vi "Text control 2 v0.1.vi"() -> ()   [LabVIEW 2013]
panel:
  out "Ion vs time":cluster{"Y data in":dbl[], "X data in":dbl[]}[](graph)
  out "Ig":dbl format="%.2e"
  out "Id":dbl format="%.2e"
  out "Is":dbl format="%.2e"
  out "I vs Vg":cluster{"Y data in":dbl[], "X data in":dbl[]}[](graph)
  in  "Suffix":string=".txt"
  in  "Prefix":string="-transfer-"
  in  "Panel Controls 2":T1={"Emergency Stop"=refnum, "TransGraph Max"=1e-05, "Text/Graph (text=false)"=TRUE, "TransGraph Min"=1e-11} {"TransGraph Min" format="%.2e"; "TransGraph Max" format="%.2e"}
  out "Currently running:":string="#output s 0 0 0 -0.008 0.008 0.002"
  in  "Lines left to run:":string
  in  "Standby":T2
  in  "Full Reset":bool
  in  "SMU4":cluster{"on/off":bool, "Voltage":dbl} {"Voltage" min=-100.0 max=100.0 format="%.2f"}
  in  "Source/Drain\nRange":u8(slide)=6 max=11 scale=0.0..11.0
  in  "Source/Drain\nRange mode":u16(ring) items=["Auto", "Limited", "Fixed"]
  in  "Gate Range":u8(slide)=6 max=11 scale=0.0..11.0
  in  "Gate Range\nmode":u16(ring) items=["Auto", "Limited", "Fixed"]
  in  "Gate":T3={"Gate Start"=0.0, "Gate Stop"=2.0, "Gate Step (linear only)"=1.0, "Gate Compliance"=0.0001, "Gate PComp"=0.0, "Range mode"=0, "Range"=6} {"Range" max=11 scale=0.0..11.0; "Range mode" items=["Auto", "Limited", "Fixed"]; "Gate PComp" format="%^.2e"; "Gate Compliance" format="%^.2e"; "Gate Step (linear only)" format="%^.4e"; "Gate Stop" format="%^.4e"; "Gate Start" format="%^.4e"}
  in  "Drain 2":T4={"Drain Start"=0.0, "Drain Stop"=2.0, "Drain Compliance"=0.0001, "Drain Step"=1.0, "Drain PComp"=0.0, "Range mode"=0, "Range"=6} {"Range" max=11 scale=0.0..11.0; "Range mode" items=["Auto", "Limited", "Fixed"]; "Drain PComp" format="%^.2e"; "Drain Step" format="%^.4e"; "Drain Compliance" format="%^.2e"; "Drain Stop" format="%^.4e"; "Drain Start" format="%^.4e"}
  in  "Timings 2":T5={"integration time"=0, "Short/Long integration time"=0.00064, "hold time (sec)"=0.0, "delay time (sec)"=0.0, "Step Time (0 disables)"=0.0, "sweep method"=0, "Pulse period"=0.005, "Base voltage"=0.0, "Pulse width"=0.0005} {"Pulse width" min=0.0005 max=0.1 step=0.0001 format="%.4f"; "Base voltage" format="%^.4e"; "Pulse period" min=0.005 max=1.0 step=0.0001 format="%.4f"; "sweep method" items=["Continuous", "Pulsed"]; "Step Time (0 disables)" format="%.2f"; "delay time (sec)" format="%.4f"; "hold time (sec)" format="%.4f"; "Short/Long integration time" format="%^.0e"; "integration time" scale=0.0..2.0}
  in  "Panel Controls":T6={"Emergency Stop"=refnum, "TransGraph Max"=1e-05, "Text/Graph (text=false)"=TRUE} {"TransGraph Max" format="%.2e"}
  in  "Interrupt run":bool
  in  "Drain: Compliance":dbl=0.001 format="%.8f"
  in  "Gate: Compliance":dbl=0.001 format="%.8f"
  out "Path":path=path "C:/users/rlp38/09Apr2009LTtesting/test2.txt"
  in  "hold time /s":dbl format="%.2f"
  in  "delay time /s":dbl format="%.2f"
  in  "integration time":u32(slide) max=2 step=1 scale=0.0..2.0
  in  "Integration time (short)":dbl=0.0019 min=8e-05 max=0.0019 step=8e-05 format="%^.0e"
  in  "Integration time (long)":dbl=0.32 min=0.04 max=2.0 step=0.02 format="%.2f"
  in  "Step delay /s":dbl format="%.2f"
  in  "Program":string="#pulsedstressV d 0.03 20 0 0.5 0.0827 5\n#\n#itime m\n#gaterangemode a\n#drainrangemode a\n#pulsed on 0.05 0 0.02\n#transfer d -10 40 1 5 40 35\n#transfer d -10 40 1 5 40 35\n#transfer d -10 40 1 5 40 35\n#output d 0 40 20 0 40 1\n#\n#\n#sample 1 0.008 221 6 0.003\n#samplei 400e-6 200 6 0.002 0.1\n#vsu2pulse -10 4\n#\n#stressV 0.016 0.03 2e-4 0.1e-3 11\n#stressI 220e-7 0.08 15\n#transfer s -1 1 0.5 -0.005 0.005 0.005\n#output s 0 0 0 -0.008 0.008 0.002\n"
  # "Syntax:\nitime [s|m|l]\ngaterangemode [a|l|f]\ndrainrangemode [a|l|f]\npulsed [on|off] PulsePeriod(sec) PulseBaseVoltage PulseONWidth(sec)\nstandby [on l off]\nwait NumMilliseconds\nwait-min NumMinutes\n# texthere = comment\ntransfer [s|d] VgStart VgStop VgStep VdStart VdStop VdStep\noutput [s|d] VgStart VgStop VgStep VdStart VdStop VdStep\nsample Vg Vd NumSamples Time(s) SampleInterval(s)\nsamplei Idg NumSamples Time(s) SampleInterval(s) VDGcompliance\n# if in doubt use SampleInterval(s) = 0.004\nstressV VG VD IGcompliance IDcompliance Duration(sec)\nstressI IDG VDGcompliance Duration(sec)\nvsu2pulse Bias Duration(s)\npulsedstressV [s|d] VEstop VgON VgOFF Period(s) PulseONwidth(s) Vd\nsample-fpp Vg Vd NumSamples Time\nresample-fpp Vg Vd\ntransfer-fpp [s|d] VgStart VgStop VgStep VdStart VdStop VdStep\noutput-fpp [s|d] VgStart VgStop VgStep VdStart VdStop VdStep"
  # "100 samples is approx 13s with medium integration"
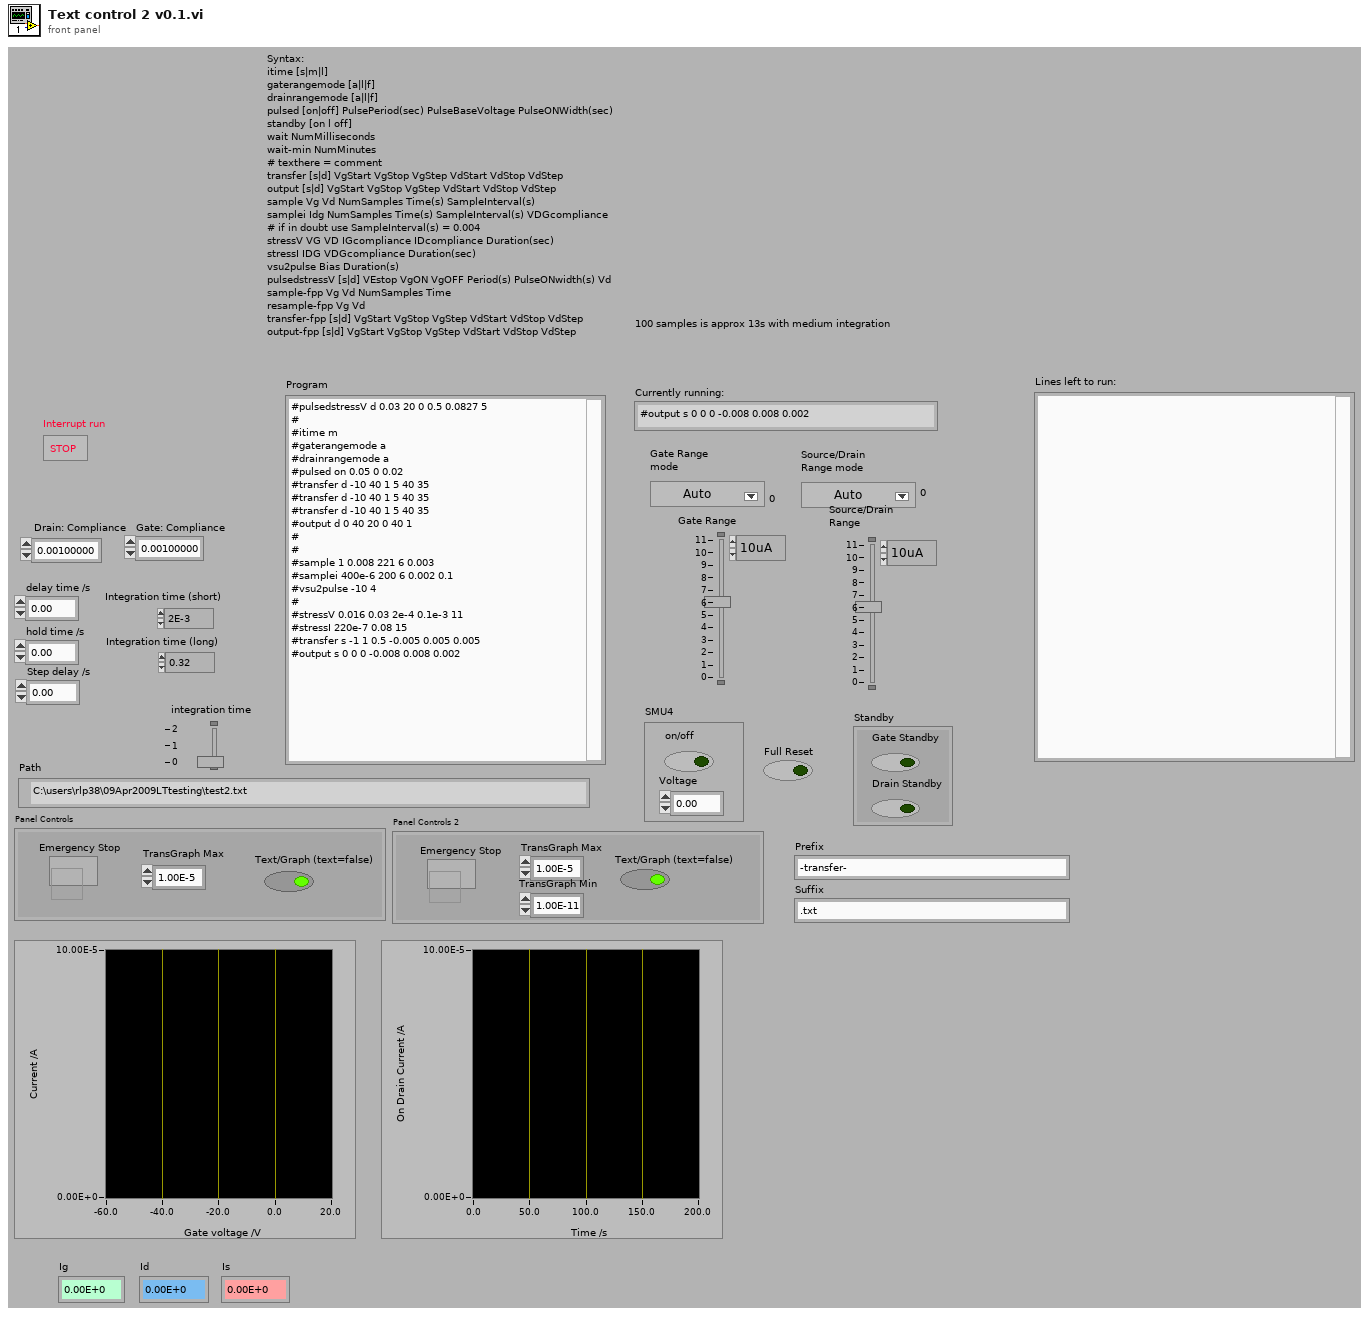
[diagram p1: front panel]
types:
  T1 = cluster{"Emergency Stop":refnum<vi>, "TransGraph Max":dbl, "Text/Graph (text=false)":bool, "TransGraph Min":dbl}
  T2 = cluster{"Gate Standby":bool, "Drain Standby":bool}
  T3 = cluster{"Gate Start":dbl, "Gate Stop":dbl, "Gate Step (linear only)":dbl, "Gate Compliance":dbl, "Gate PComp":dbl, "Range mode":u16, "Range":u8}
  T4 = cluster{"Drain Start":dbl, "Drain Stop":dbl, "Drain Compliance":dbl, "Drain Step":dbl, "Drain PComp":dbl, "Range mode":u16, "Range":u8}
  T5 = cluster{"integration time":u32, "Short/Long integration time":dbl, "hold time (sec)":dbl, "delay time (sec)":dbl, "Step Time (0 disables)":dbl, "sweep method":u16, "Pulse period":dbl, "Base voltage":dbl, "Pulse width":dbl}
  T6 = cluster{"Emergency Stop":refnum<vi>, "TransGraph Max":dbl, "Text/Graph (text=false)":bool}
  T7 = enum16{"open", "replace", "create", "open or create", "replace or create", "replace or create with confirmation"}
  T8 = cluster{"V2 Start":dbl, "V2 Step":dbl, "Number of points":i32}
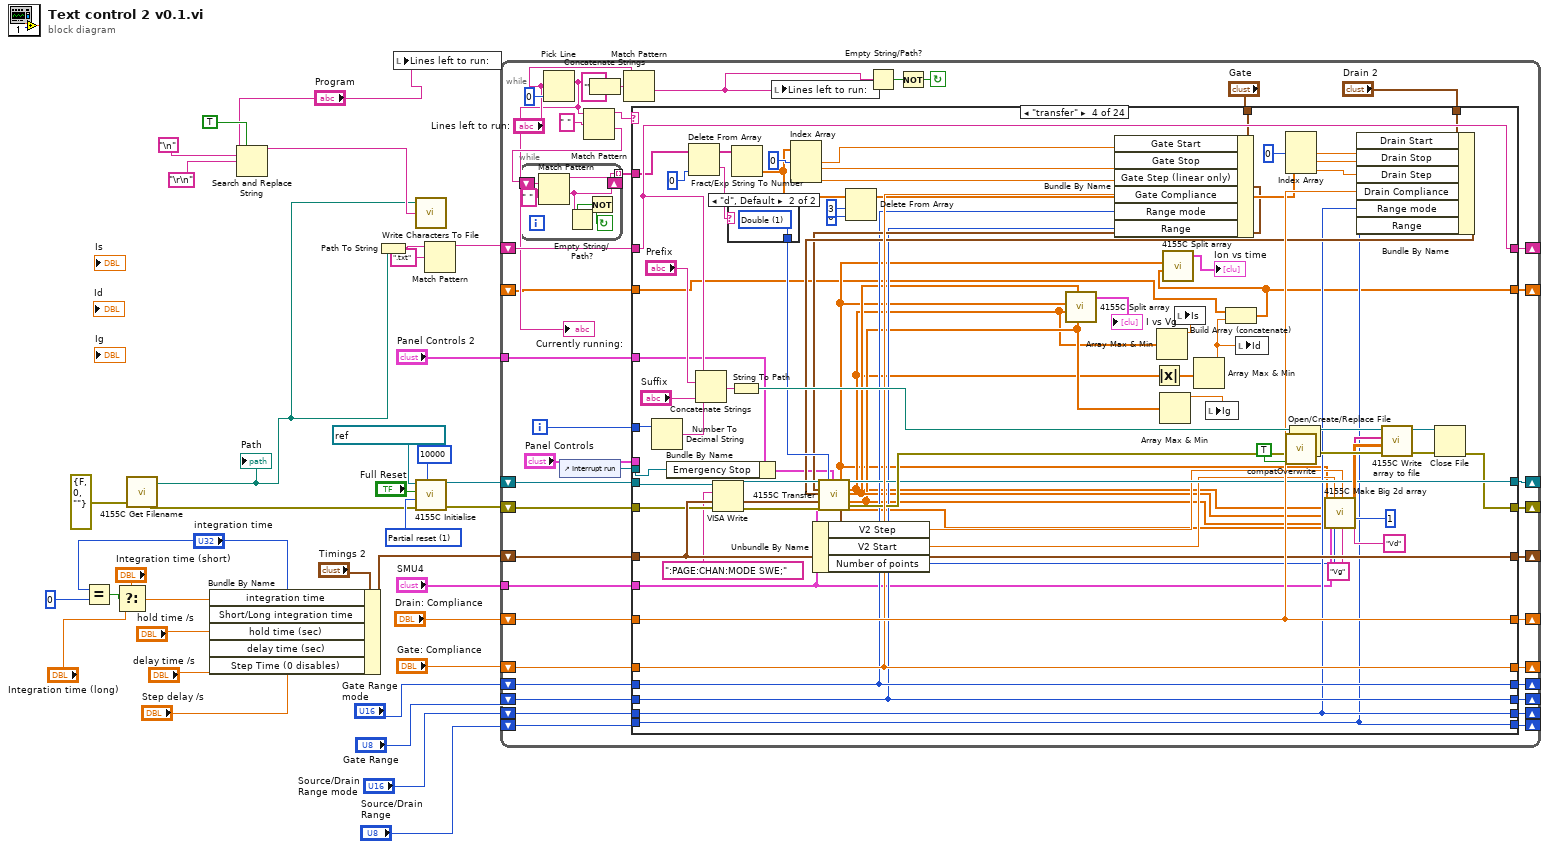
[diagram p0: block diagram]
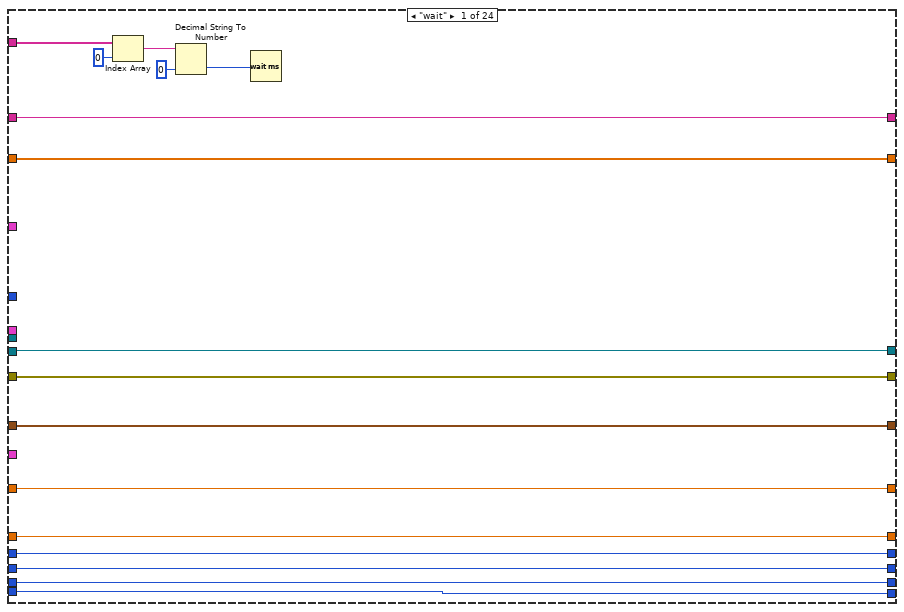
[diagram p2: hidden frame]
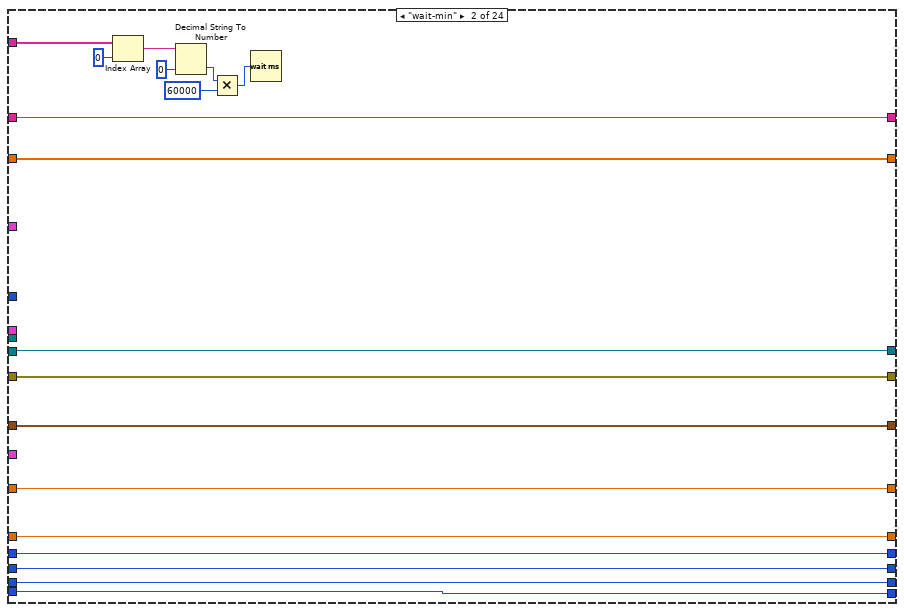
[diagram p3: hidden frame]
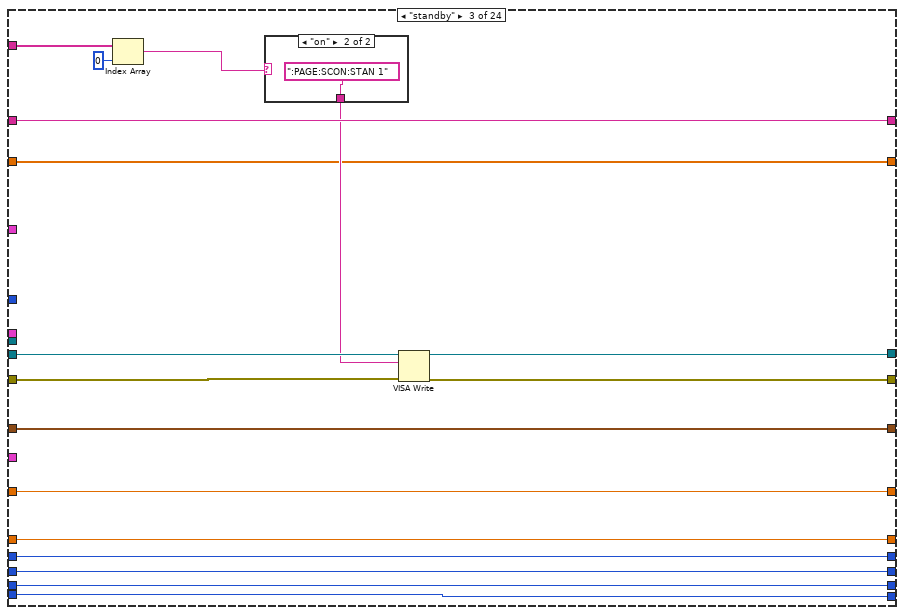
[diagram p4: hidden frame]
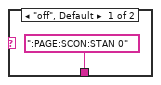
[diagram p5: hidden frame]
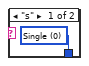
[diagram p6: hidden frame]
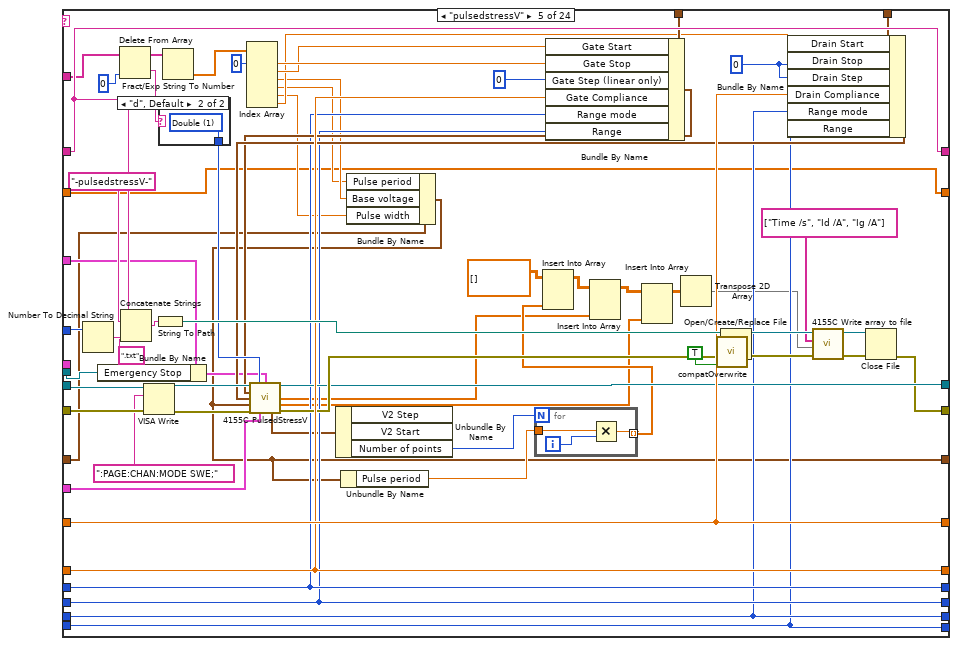
[diagram p7: hidden frame]
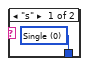
[diagram p8: hidden frame]
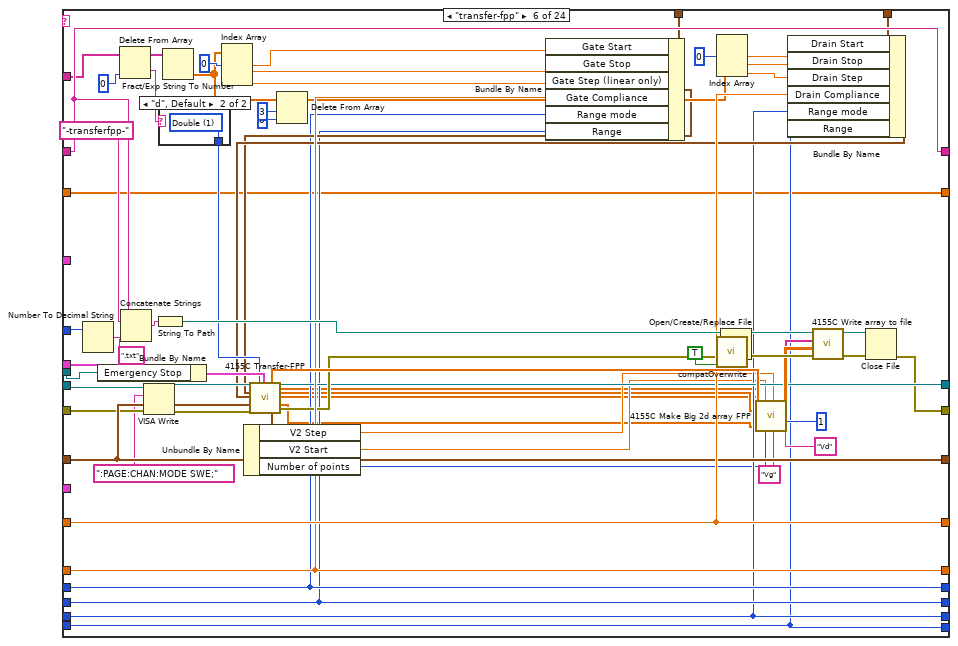
[diagram p9: hidden frame]
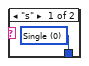
[diagram p10: hidden frame]
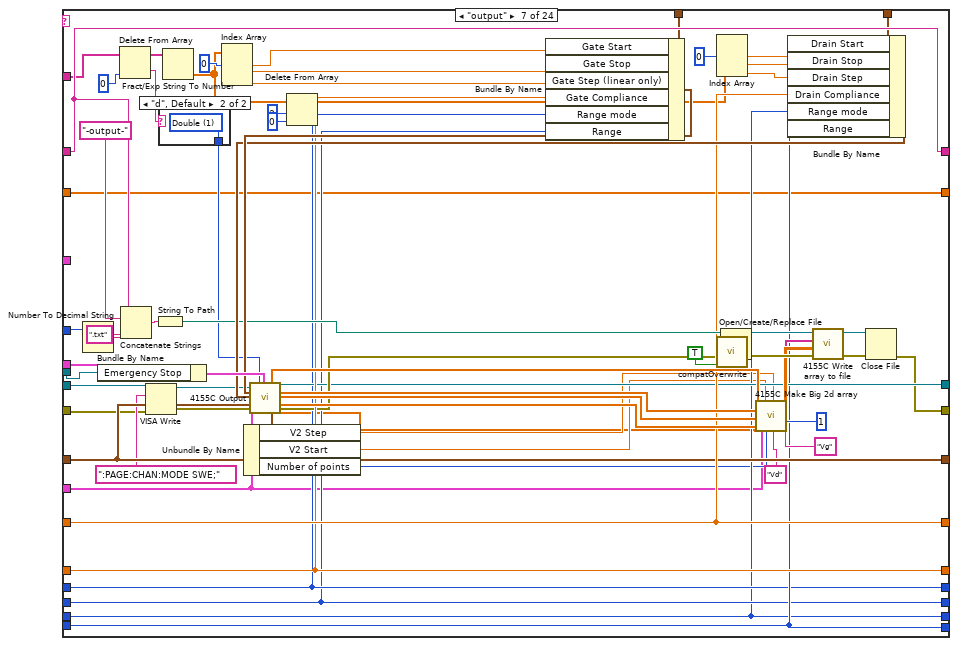
[diagram p11: hidden frame]
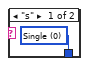
[diagram p12: hidden frame]
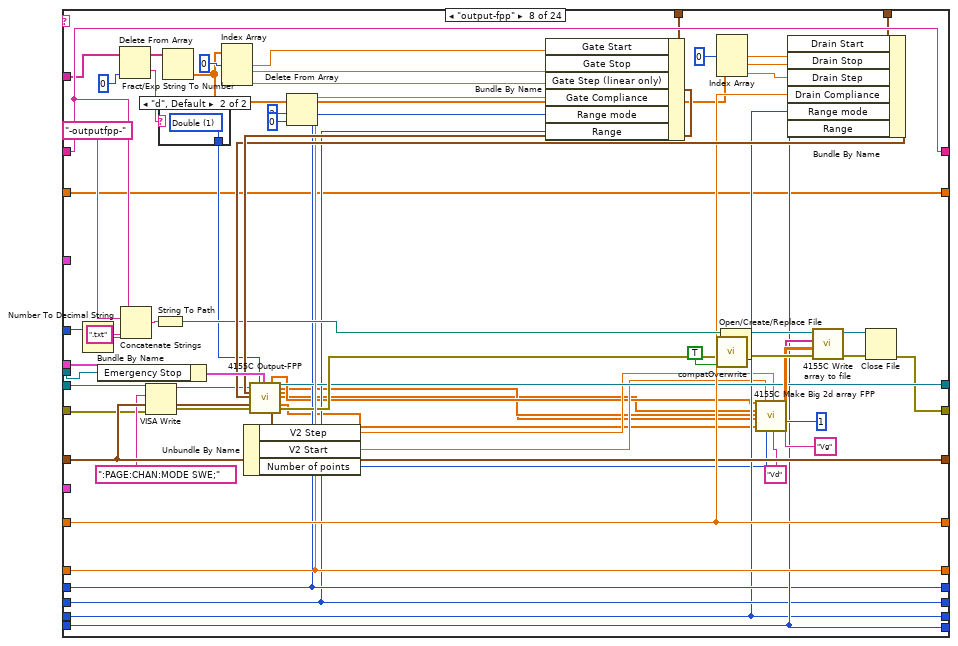
[diagram p13: hidden frame]
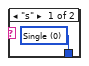
[diagram p14: hidden frame]
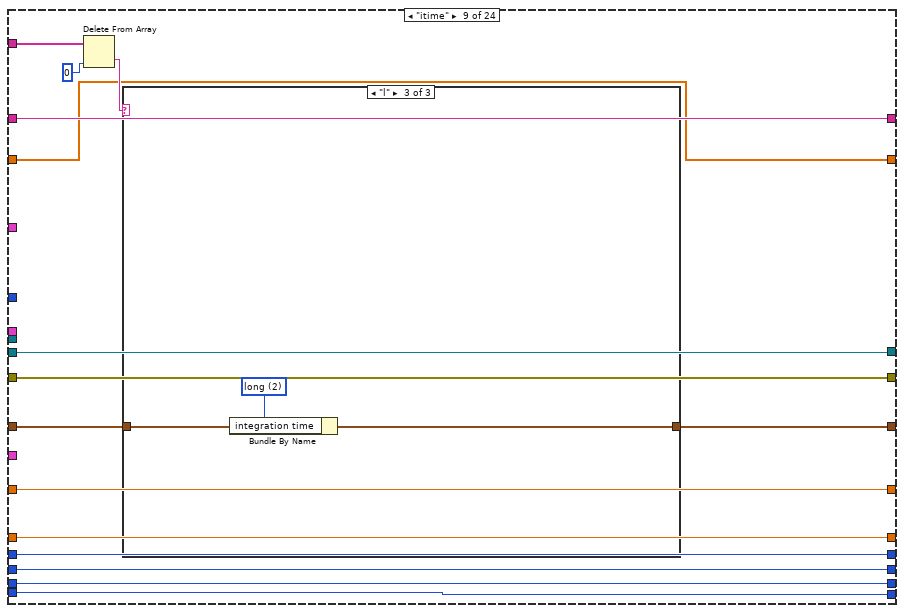
[diagram p15: hidden frame]
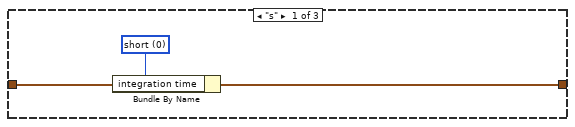
[diagram p16: hidden frame]
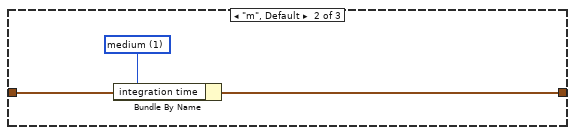
[diagram p17: hidden frame]
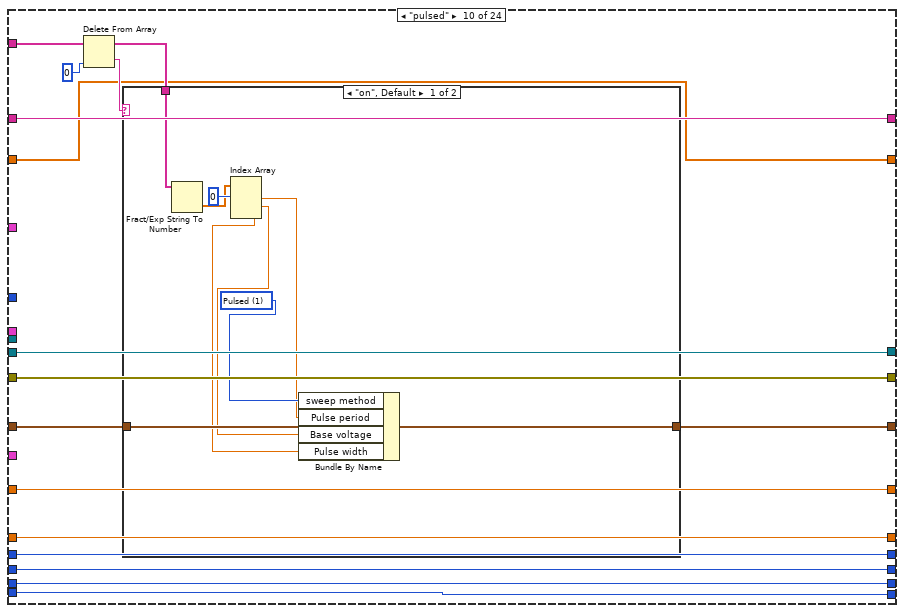
[diagram p18: hidden frame]
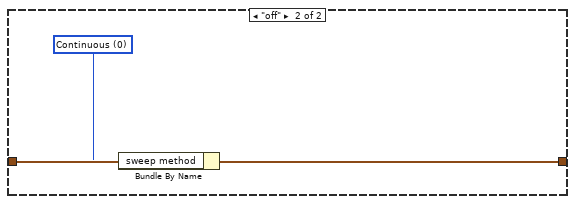
[diagram p19: hidden frame]
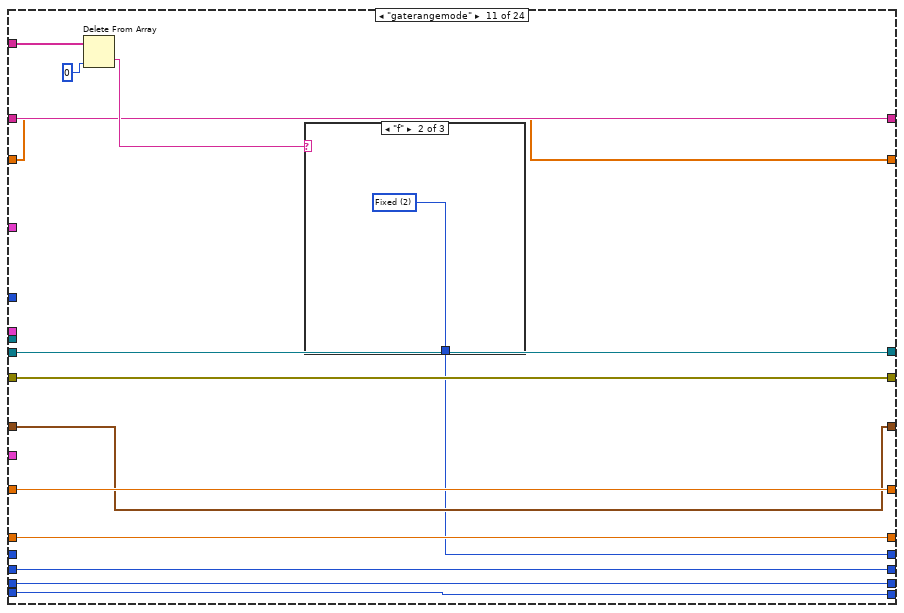
[diagram p20: hidden frame]
diagram:
  w27 = u16 1 items=["Reset All", "Partial reset"] ("Type of reset")
  n1 = Equal?(x="integration time", y=u32 0) -> (x = y?=w31:bool)
  n2 = Select(t="Integration time (short)", s=w31, f="Integration time (long)") -> (s? t:f=w35:dbl)
  n3 = call <userlib>:"4155C Get Filename.vi"("error in (no error)"=errorcluster {"status"=FALSE, "code"=0, "source"=""}) -> ("error out"=w22:errorcluster, "path"=w6:path)  [unwired: 2 in, 1 out]
  "Path" <- w6
  n4 = Bundle By Name(cluster="Timings 2", "integration time"="integration time", "Short/Long integration time"=w35, "hold time (sec)"="hold time /s", "delay time (sec)"="delay time /s", "Step Time (0 disables)"="Step delay /s") -> (w19:T5)
  n5 = Search and Replace String(replace all?=TRUE ("replace all? (F)"), input string="Program", search string="\n", replace string="\r\n") -> (result string=w9:string)  [unwired: 4 in, 3 out]
  n6 = Path To String(path=w6) -> (string=w5:string)
  n7 = local write "Lines left to run:"("Program") -> ()
  n8 = call <vilib>:"Write Characters To File.vi"("character string"=w9, "file path (dialog if empty)"=w6) -> ()  [unwired: 3 in, 1 out]
  n9 = call <userlib>:"4155C Initialise.vi"("VISA resource name in"=refnum<visa-resource-name> "GPIB0::14::INSTR", "Reset"="Full Reset", "Type of reset"=w27, "error in (no error)"=w22, "VISA Timeout Value"=u32 10000) -> ("VISA Resource Name out"=w21:refnum<visa-resource-name>, "error out"=w20:errorcluster)
  n10 = Match Pattern(string=w5, regular expression=".txt") -> (before substring=w4:string)  [unwired: 1 in, 3 out]
  n11 = while {
    tunnel: "SMU4" -> [w43]
    shift-left: "Source/Drain\nRange" -> [w48]
    shift-right: [w44] -> _
    shift-left: "Source/Drain\nRange mode" -> [w49]
    shift-right: [w45] -> _
    shift-left: "Gate Range" -> [w50]
    shift-right: [w46] -> _
    shift-left: "Gate Range\nmode" -> [w51]
    shift-right: [w47] -> _
    shift-left: "Gate: Compliance" -> [w63]
    shift-right: [w57] -> _
    shift-left: "Drain: Compliance" -> [w64]
    shift-right: [w58] -> _
    shift-left: w19 -> [w65]
    shift-right: [w59] -> _
    shift-left: w20 -> [w66]
    shift-right: [w60] -> _
    shift-left: w21 -> [w67]
    shift-right: [w61] -> _
    shift-left: w4 -> [w68]
    shift-right: [w56] -> _
    tunnel: "Panel Controls 2" -> [w39]
    shift-right: [w38] -> _
    shift-left: _ -> [w37]
    i -> [w62]
    stop <- w76 continue-if-true
    n12 = Pick Line(multi-line string="Lines left to run:", line index=0) -> (output string=w40:string)  [unwired: 1 in]
    "Currently running:" <- w40
    n13 = control-ref of="Interrupt run"() -> (w55:refnum<vi>)
    n14 = Match Pattern(string=w40, regular expression=" ") -> (before substring=w71:string, after substring=w70:string)  [unwired: 1 in, 2 out]
    n15 = while {
      tunnel: [w78] -> w69 mode=indexing
      shift-left: w70 -> [w80]
      shift-right: [w79] -> _
      stop <- w82 continue-if-true
      n16 = Match Pattern(string=w80, regular expression=" ") -> (before substring=w78:string, after substring=w79:string)  [unwired: 1 in, 2 out]
      n17 = Empty String/Path?(string/path=w79) -> (empty?=w83:bool)
      n18 = Not(x=w83) -> (.not. x?=w82:bool)
    }
    n19 = Concatenate Strings(w40, "\n" ("Substring")) -> (w74:string)
    n20 = Match Pattern(string="Lines left to run:", regular expression=w74) -> (after substring=w41:string)  [unwired: 1 in, 3 out]
    n21 = case shown="\"transfer\"" w71 {
      tunnel: w69 -> [w99 w117 w134 w191 w261 w328 w393 w466 w504 w529 w555 w579 w599 w612 _ _ w710 w769 _ w831 w873 w913 w981 w1041]
      tunnel: w68 -> [w94 w113 w132 w199 w268 w336 w401 w474 w493 w518 w547 w572 w593 w605 w623 w662 w688 w751 w782 w818 w860 w901 w975 w1037]
      tunnel: w67 -> [w93 w112 w123 w169 w252 w305 w369 w442 w494 w519 w548 w573 w594 w606 w628 w665 w717 w776 w786 w838 w880 w920 w988 w994]
      tunnel: w66 -> [w92 w111 w122 w168 w251 w304 w366 w439 w495 w520 w549 w574 w595 w607 w627 w634 w716 w775 w785 w837 w879 w919 w987 w993]
      tunnel: w65 -> [w91 w110 w131 w195 w226 w332 w397 w470 w503 w528 w546 w571 w592 w604 w626 w658 w679 w743 w791 w811 w853 w894 w974 w1036]
      tunnel: w64 -> [w90 w109 w130 w197 w266 w334 w399 w472 w502 w527 w554 w578 w598 w611 w625 w643 w715 w774 w794 w836 w878 w918 w986 w1046]
      tunnel: w63 -> [w89 w108 w129 w196 w265 w333 w398 w471 w501 w526 w553 w577 w597 w610 w624 w644 w689 w752 w793 w819 w861 w902 w976 w1038]
      tunnel: w62 -> [_ _ _ w200 w269 w337 w402 w475 _ _ _ _ _ _ _ w660 w714 w773 _ w835 w877 w917 w985 w1045]
      tunnel: [w93 w112 w121 w193 w263 w330 w395 w468 w494 w519 w548 w573 w594 w606 w628 w665 w680 w724 w784 w812 w854 w895 w926 w996] -> w61
      tunnel: [w92 w111 w120 w192 w262 w329 w394 w467 w495 w520 w549 w574 w595 w607 w627 w633 w690 w725 w783 w820 w862 w903 w925 w995] -> w60
      tunnel: [w91 w110 w131 w195 w222 w332 w397 w470 w496 w521 w546 w571 w592 w604 w626 w658 w679 w743 w791 w811 w853 w894 w974 w1036] -> w59
      tunnel: [w90 w109 w130 w197 w266 w334 w399 w472 w502 w527 w554 w578 w598 w611 w625 w643 w715 w774 w794 w836 w878 w918 w986 w1046] -> w58
      tunnel: [w89 w108 w129 w196 w265 w333 w398 w471 w501 w526 w553 w577 w597 w610 w624 w644 w689 w752 w793 w819 w861 w902 w976 w1038] -> w57
      tunnel: [w94 w113 w132 w199 w268 w336 w401 w474 w493 w518 w547 w572 w593 w605 w623 w662 w688 w751 w782 w818 w860 w901 w975 w1037] -> w56
      tunnel: w55 -> [_ _ _ w204 w273 w342 w410 w479 _ _ _ _ _ _ _ _ w685 w748 _ w817 w859 w900 w946 w1012]
      tunnel: "Gate" -> [_ _ _ w178 w255 w315 w380 w453 _ _ _ _ _ _ _ _ _ _ _ _ _ _ _ _]
      tunnel: "Drain 2" -> [_ _ _ w177 w254 w314 w379 w452 _ _ _ _ _ _ _ _ _ _ _ _ _ _ _ _]
      tunnel: "Panel Controls" -> [_ _ _ _ _ w313 w378 w451 _ _ _ _ _ _ _ _ _ _ _ _ _ _ _ _]
      tunnel: w51 -> [w88 w107 w128 w162 w245 w298 w364 w437 w500 w525 _ w570 w591 w603 w622 w645 w675 w739 w787 w807 w849 w890 w970 w1032]
      tunnel: w50 -> [w87 w106 w127 w161 w244 w297 w363 w436 w499 w524 w552 _ w582 w609 w621 w646 w676 w740 w788 w808 w850 w891 w971 w1033]
      tunnel: w49 -> [w86 w105 w126 w160 w243 w296 w362 w435 w498 w523 w551 w576 w596 _ w620 w647 w677 w741 w789 w809 w851 w892 w972 w1034]
      tunnel: w48 -> [w85 w104 w125 w159 w242 w295 w365 w438 w497 w522 w550 w575 _ w608 w619 w648 w678 w742 w790 w810 w852 w893 w973 w1035]
      tunnel: [w88 w107 w128 w162 w245 w298 w364 w437 w500 w525 w545 w570 w591 w603 w622 w645 w675 w739 w787 w807 w849 w890 w970 w1032] -> w47
      tunnel: [w87 w106 w127 w161 w244 w297 w363 w436 w499 w524 w552 w562 w582 w609 w621 w646 w676 w740 w788 w808 w850 w891 w971 w1033] -> w46
      tunnel: [w86 w105 w126 w160 w243 w296 w362 w435 w498 w523 w551 w576 w596 w602 w620 w647 w677 w741 w789 w809 w851 w892 w972 w1034] -> w45
      tunnel: [w85 w104 w125 w159 w242 w295 w365 w438 w497 w522 w550 w575 w583 w608 w619 w648 w678 w742 w790 w810 w852 w893 w973 w1035] -> w44
      tunnel: w43 -> [_ _ _ w152 w238 _ w356 _ _ _ _ _ _ _ _ _ _ _ _ _ _ _ _ _]
      tunnel: w39 -> [_ _ _ w150 w237 _ _ _ _ _ _ _ _ _ _ _ _ _ _ _ _ _ _ _]
      tunnel: [w84 w100 w118 w138 w214 w284 w353 w423 w492 w516 w544 w561 w581 w601 w618 w629 w666 w722 w781 w795 w841 w883 w923 w989] -> w38
      tunnel: w37 -> [w84 w100 w118 w137 w214 w284 w353 w423 w492 w516 w544 w561 w581 w601 w618 w629 w666 w722 w781 w795 w841 w883 w923 w989]
      frame "wait" {
        n22 = Index Array(array=w99, index=0 ("Index")) -> (element=w97:string)
        n23 = Decimal String To Number(string=w97, default (0L)=u32 0) -> (number=w96:u32)  [unwired: 1 in, 1 out]
        n24 = Wait (ms)(milliseconds to wait=w96) -> ()  [unwired: 1 out]
      }
      frame "wait-min" {
        n25 = Index Array(array=w117, index=0 ("Index")) -> (element=w115:string)
        n26 = Decimal String To Number(string=w115, default (0L)=u32 0) -> (number=w103:u32)  [unwired: 1 in, 1 out]
        n27 = Multiply(x=w103, y=u32 60000) -> (x*y=w102:u32)
        n28 = Wait (ms)(milliseconds to wait=w102) -> ()  [unwired: 1 out]
      }
      frame "standby" {
        n29 = Index Array(array=w134, index=0 ("Index")) -> (element=w124:string)
        n30 = case shown="\"on\"" w124 {
          tunnel: [":PAGE:SCON:STAN 0" ":PAGE:SCON:STAN 1"] -> w119
          frame "off", Default {
          }
          frame "on" {
          }
        }
        n31 = VISA Write(VISA resource name=w123, write buffer=w119, error in (no error)=w122) -> (VISA resource name out=w121:refnum<visa-resource-name>, error out=w120:errorcluster)  [unwired: 1 out]
      }
      frame "transfer" {
        n32 = Number To Decimal String(number=w200) -> (decimal integer string=w201:string)  [unwired: 1 in]
        n33 = Bundle By Name(cluster=w150, "Emergency Stop"=w204) -> (w151:T1)
        n34 = Delete From Array(array=w191, index=0 ("Index")) -> (deleted portion=w189:string, array with subset deleted=w188:string[])  [unwired: 1 in]
        n35 = Concatenate Strings(w199, "Prefix", w201, "Suffix") -> (w203:string)
        n36 = VISA Write(VISA resource name=w169, write buffer=":PAGE:CHAN:MODE SWE;" ("write buffer (\"\")"), error in (no error)=w168) -> (VISA resource name out=w166:refnum<visa-resource-name>, error out=w167:errorcluster)  [unwired: 1 out]
        n37 = case shown="\"d\", Default" w189 {
          tunnel: [w212 w213] -> w187
          frame "s" {
            w212 = u16 0 items=["Single", "Double"] ("sweep mode")
          }
          frame "d", Default {
            w213 = u16 1 items=["Single", "Double"] ("sweep mode")
          }
        }
        n38 = String To Path(string=w203) -> (path=w198:path)
        n39 = Fract/Exp String To Number(string=w188) -> (number=w173:dbl[])  [unwired: 3 in, 1 out]
        n40 = Index Array(array=w173, index #1=0 ("Index")) -> (element #1=w186:dbl, element #2=w185:dbl, element #3=w184:dbl)  [unwired: 2 in]
        n41 = Delete From Array(array=w173, length=3 ("Length"), index=0 ("Index")) -> (array with subset deleted=w171:dbl[])  [unwired: 1 out]
        n42 = Bundle By Name(cluster=w178, "Gate Start"=w186, "Gate Stop"=w185, "Gate Step (linear only)"=w184, "Gate Compliance"=w196, "Range mode"=w162, "Range"=w161) -> (w163:T3)
        n43 = Index Array(array=w171, index #1=0 ("Index")) -> (element #1=w181:dbl, element #2=w180:dbl, element #3=w179:dbl)  [unwired: 2 in]
        n44 = call <vilib>:"compatOverwrite.vi"("overwrite (F)"=TRUE) -> ("overwrite?"=w149:T7)
        n45 = Bundle By Name(cluster=w177, "Drain Start"=w181, "Drain Stop"=w180, "Drain Step"=w179, "Drain Compliance"=w197, "Range mode"=w160, "Range"=w159) -> (w164:T4)
        n46 = call <userlib>:"4155C Transfer.vi"("VISA resource name in"=w166, "Gate"=w163, "Drain"=w164, "Timings"=w195, "error in (no error)"=w167, "SMU4"=w152, "sweep mode"=w187, "Panel Controls"=w151) -> ("VG"=w140:dbl[], "Outparams"=w157:T8, "VISA Resource Name out"=w193:refnum<visa-resource-name>, "IS"=w142:dbl[], "ID"=w147:dbl[], "IG"=w143:dbl[], "error out"=w194:errorcluster, "SMU4"=w153:dbl[])  [unwired: 12 in]
        n47 = Unbundle By Name(w157) -> ("V2 Step"=w156:dbl, "V2 Start"=w155:dbl, "Number of points"=w154:i32)
        n48 = call <userlib>:"4155C Split array.vi"("Y2 data in"=w147, "X data in"=w140, "Y1 data in"=w142, "Y3 data in"=w143) -> ("Array of clusters"=→"I vs Vg":cluster{"Y data in":dbl[], "X data in":dbl[]}[])  [unwired: 3 in, 1 out]
        n49 = Absolute Value(x=w142) -> (abs(x)=w146:dbl[])
        n50 = Array Max & Min(array=w142) -> (max value=w144:dbl)  [unwired: 3 out]
        n51 = Array Max & Min(array=w143) -> (max value=w145:dbl)  [unwired: 3 out]
        n52 = local write "Is"(w144) -> ()
        n53 = Array Max & Min(array=w146) -> (max value=w139:dbl)  [unwired: 3 out]
        n54 = local write "Ig"(w145) -> ()
        n55 = Build Array (concatenate)(w137, w139) -> (w138:dbl[])
        n56 = call <userlib>:"4155C Split array.vi"("X data in"=w140, "Y1 data in"=w138) -> ("Array of clusters"=→"Ion vs time":cluster{"Y data in":dbl[], "X data in":dbl[]}[])  [unwired: 5 in, 1 out]
        n57 = local write "Id"(w139) -> ()
        n58 = Open/Create/Replace File(file path (use dialog)=w198, error in=w194, operation (0:open)=w149) -> (refnum out=w209:refnum<file>, error out=w210:errorcluster)  [unwired: 3 in, 1 out]
        n59 = call <userlib>:"4155C Make Big 2d array.vi"("1D Var1"=w140, "1d IS"=w142, "1d ID"=w147, "1d IG"=w143, "1d SMU4"=w153, "SMU4"=w152, "VAR2 START"=w155, "Number of VAR2 steps"=w154, "VAR2 STEP"=w156, "VAR1 Name"="Vg", "Decimal places in header"=i8 1, "VAR2 Name"="Vd") -> ("Header array"=w205:string[], "Data array"=w206:dbl[][])  [unwired: 14 in]
        n60 = call <userlib>:"4155C Write array to file.vi"("Byte Stream File Refnum"=w209, "Header"=w205, "Data Array"=w206, "error in (no error)"=w210) -> ("dup refnum"=w207:refnum<file>, "error out"=w208:errorcluster)  [unwired: 1 in]
        n61 = Close File(refnum=w207, error in=w208) -> (error out=w192:errorcluster)  [unwired: 1 out]
      }
      frame "pulsedstressV" {
        w220 = 0
        n62 = Number To Decimal String(number=w269) -> (decimal integer string=w270:string)  [unwired: 1 in]
        n63 = Bundle By Name(cluster=w237, "Emergency Stop"=w273) -> (w239:T1)
        n64 = Delete From Array(array=w261, index=0 ("Index")) -> (deleted portion=w259:string, array with subset deleted=w258:string[])  [unwired: 1 in]
        n65 = Concatenate Strings(w268, "-pulsedstressV-" ("Substring"), w270, ".txt" ("Substring")) -> (w272:string)
        n66 = VISA Write(VISA resource name=w252, write buffer=":PAGE:CHAN:MODE SWE;" ("write buffer (\"\")"), error in (no error)=w251) -> (VISA resource name out=w249:refnum<visa-resource-name>, error out=w250:errorcluster)  [unwired: 1 out]
        n67 = String To Path(string=w272) -> (path=w267:path)
        n68 = case shown="\"d\", Default" w259 {
          tunnel: [w282 w283] -> w257
          frame "s" {
            w282 = u16 0 items=["Single", "Double"] ("sweep mode")
          }
          frame "d", Default {
            w283 = u16 1 items=["Single", "Double"] ("sweep mode")
          }
        }
        n69 = Fract/Exp String To Number(string=w258) -> (number=w253:dbl[])  [unwired: 3 in, 1 out]
        n70 = Index Array(array=w253, index #1=0 ("Index")) -> (element #1=w229:dbl, element #2=w228:dbl, element #3=w225:dbl, element #4=w224:dbl, element #5=w223:dbl, element #6=w227:dbl)  [unwired: 5 in]
        n71 = Bundle By Name(cluster=w226, "Pulse period"=w224, "Base voltage"=w225, "Pulse width"=w223) -> (w222:T5)
        n72 = Unbundle By Name(w222) -> ("Pulse period"=w230:dbl)
        n73 = Bundle By Name(cluster=w255, "Gate Start"=w228, "Gate Stop"=w229, "Gate Step (linear only)"=0, "Gate Compliance"=w265, "Range mode"=w245, "Range"=w244) -> (w246:T3)
        n74 = call <vilib>:"compatOverwrite.vi"("overwrite (F)"=TRUE) -> ("overwrite?"=w215:T7)
        n75 = Bundle By Name(cluster=w254, "Drain Start"=w227, "Drain Stop"=w220, "Drain Step"=w220, "Drain Compliance"=w266, "Range mode"=w243, "Range"=w242) -> (w247:T4)
        n76 = call <userlib>:"4155C PulsedStressV.vi"("VISA resource name in"=w249, "sweep mode"=w257, "Panel Controls"=w239, "Gate"=w246, "Drain"=w247, "Timings"=w222, "error in (no error)"=w250, "SMU4"=w238) -> ("VISA Resource Name out"=w263:refnum<visa-resource-name>, "ID"=w218:dbl[], "IG"=w216:dbl[], "Outparams"=w240:T8, "error out"=w264:errorcluster)  [unwired: 3 in]
        n77 = Unbundle By Name(w240) -> ("Number of points"=w217:i32)  [unwired: 2 out]
        n78 = for {
          N: w217 -> [_]
          tunnel: [w279] -> w219 mode=indexing
          tunnel: w230 -> [w281]
          i -> [w280]
          n79 = Multiply(x=w281, y=w280) -> (x*y=w279:dbl)
        }
        n80 = Insert Into Array(array=dbl[][] [] ("Input Array"), new element=w219) -> (w231:dbl[][])  [unwired: 2 in]
        n81 = Insert Into Array(array=w231, new element=w218) -> (w236:dbl[][])  [unwired: 2 in]
        n82 = Insert Into Array(array=w236, new element=w216) -> (w235:dbl[][])  [unwired: 2 in]
        n83 = Transpose 2D Array(2D array=w235) -> (transposed array=w234:dbl[][])
        n84 = Open/Create/Replace File(file path (use dialog)=w267, error in=w264, operation (0:open)=w215) -> (refnum out=w276:refnum<file>, error out=w277:errorcluster)  [unwired: 3 in, 1 out]
        n85 = call <userlib>:"4155C Write array to file.vi"("Byte Stream File Refnum"=w276, "Header"=string[] ["Time /s", "Id /A", "Ig /A"], "Data Array"=w234, "error in (no error)"=w277) -> ("dup refnum"=w274:refnum<file>, "error out"=w275:errorcluster)  [unwired: 1 in]
        n86 = Close File(refnum=w274, error in=w275) -> (error out=w262:errorcluster)  [unwired: 1 out]
      }
      frame "transfer-fpp" {
        n87 = Number To Decimal String(number=w337) -> (decimal integer string=w338:string)  [unwired: 1 in]
        n88 = Bundle By Name(cluster=w313, "Emergency Stop"=w342) -> (w350:T6)
        n89 = Delete From Array(array=w328, index=0 ("Index")) -> (deleted portion=w326:string, array with subset deleted=w325:string[])  [unwired: 1 in]
        n90 = Concatenate Strings(w336, "-transferfpp-" ("Substring"), w338, ".txt" ("Substring")) -> (w340:string)
        n91 = VISA Write(VISA resource name=w305, write buffer=":PAGE:CHAN:MODE SWE;" ("write buffer (\"\")"), error in (no error)=w304) -> (VISA resource name out=w302:refnum<visa-resource-name>, error out=w303:errorcluster)  [unwired: 1 out]
        n92 = String To Path(string=w340) -> (path=w335:path)
        n93 = case shown="\"d\", Default" w326 {
          tunnel: [w351 w352] -> w324
          frame "s" {
            w351 = u16 0 items=["Single", "Double"] ("sweep mode")
          }
          frame "d", Default {
            w352 = u16 1 items=["Single", "Double"] ("sweep mode")
          }
        }
        n94 = Fract/Exp String To Number(string=w325) -> (number=w309:dbl[])  [unwired: 3 in, 1 out]
        n95 = Index Array(array=w309, index #1=0 ("Index")) -> (element #1=w323:dbl, element #2=w322:dbl, element #3=w321:dbl)  [unwired: 2 in]
        n96 = Delete From Array(array=w309, length=3 ("Length"), index=0 ("Index")) -> (array with subset deleted=w307:dbl[])  [unwired: 1 out]
        n97 = Bundle By Name(cluster=w315, "Gate Start"=w323, "Gate Stop"=w322, "Gate Step (linear only)"=w321, "Gate Compliance"=w333, "Range mode"=w298, "Range"=w297) -> (w299:T3)
        n98 = Index Array(array=w307, index #1=0 ("Index")) -> (element #1=w318:dbl, element #2=w317:dbl, element #3=w316:dbl)  [unwired: 2 in]
        n99 = call <vilib>:"compatOverwrite.vi"("overwrite (F)"=TRUE) -> ("overwrite?"=w285:T7)
        n100 = Bundle By Name(cluster=w314, "Drain Start"=w318, "Drain Stop"=w317, "Drain Step"=w316, "Drain Compliance"=w334, "Range mode"=w296, "Range"=w295) -> (w300:T4)
        n101 = call <userlib>:"4155C Transfer-FPP.vi"("VISA resource name in"=w302, "Gate"=w299, "Drain"=w300, "Timings"=w332, "error in (no error)"=w303, "sweep mode"=w324, "Panel Controls"=w350) -> ("VG"=w341:dbl[], "Outparams"=w293:T8, "VISA Resource Name out"=w330:refnum<visa-resource-name>, "Vprobe2"=w289:dbl[], "ID"=w288:dbl[], "IG"=w287:dbl[], "Vprobe1"=w286:dbl[], "error out"=w331:errorcluster)  [unwired: 13 in]
        n102 = Unbundle By Name(w293) -> ("V2 Step"=w292:dbl, "V2 Start"=w291:dbl, "Number of points"=w290:i32)
        n103 = Open/Create/Replace File(file path (use dialog)=w335, error in=w331, operation (0:open)=w285) -> (refnum out=w347:refnum<file>, error out=w348:errorcluster)  [unwired: 3 in, 1 out]
        n104 = call <userlib>:"4155C Make Big 2d array FPP.vi"("1D Var1"=w341, "1d ID"=w288, "1d Vp2"=w289, "1d IG"=w287, "1d Vp1"=w286, "VAR2 START"=w291, "Number of VAR2 steps"=w290, "VAR2 STEP"=w292, "VAR1 Name"="Vg", "Decimal places in header"=i8 1, "VAR2 Name"="Vd") -> ("Header array"=w343:string[], "Data array"=w344:dbl[][])  [unwired: 15 in]
        n105 = call <userlib>:"4155C Write array to file.vi"("Byte Stream File Refnum"=w347, "Header"=w343, "Data Array"=w344, "error in (no error)"=w348) -> ("dup refnum"=w345:refnum<file>, "error out"=w346:errorcluster)  [unwired: 1 in]
        n106 = Close File(refnum=w345, error in=w346) -> (error out=w329:errorcluster)  [unwired: 1 out]
      }
      frame "output" {
        n107 = Number To Decimal String(number=w402) -> (decimal integer string=w403:string)  [unwired: 1 in]
        n108 = Bundle By Name(cluster=w378, "Emergency Stop"=w410) -> (w420:T6)
        n109 = Delete From Array(array=w393, index=0 ("Index")) -> (deleted portion=w391:string, array with subset deleted=w390:string[])  [unwired: 1 in]
        n110 = Concatenate Strings(w401, "-output-" ("Substring"), w403, ".txt" ("Substring")) -> (w405:string)
        n111 = VISA Write(VISA resource name=w369, write buffer=":PAGE:CHAN:MODE SWE;" ("write buffer (\"\")"), error in (no error)=w366) -> (VISA resource name out=w368:refnum<visa-resource-name>, error out=w367:errorcluster)  [unwired: 1 out]
        n112 = String To Path(string=w405) -> (path=w400:path)
        n113 = case shown="\"d\", Default" w391 {
          tunnel: [w421 w422] -> w389
          frame "s" {
            w421 = u16 0 items=["Single", "Double"] ("sweep mode")
          }
          frame "d", Default {
            w422 = u16 1 items=["Single", "Double"] ("sweep mode")
          }
        }
        n114 = Fract/Exp String To Number(string=w390) -> (number=w372:dbl[])  [unwired: 3 in, 1 out]
        n115 = Index Array(array=w372, index #1=0 ("Index")) -> (element #1=w388:dbl, element #2=w387:dbl, element #3=w386:dbl)  [unwired: 2 in]
        n116 = Delete From Array(array=w372, length=3 ("Length"), index=0 ("Index")) -> (array with subset deleted=w371:dbl[])  [unwired: 1 out]
        n117 = Bundle By Name(cluster=w380, "Gate Start"=w388, "Gate Stop"=w387, "Gate Step (linear only)"=w386, "Gate Compliance"=w398, "Range mode"=w364, "Range"=w363) -> (w419:T3)
        n118 = Index Array(array=w371, index #1=0 ("Index")) -> (element #1=w383:dbl, element #2=w382:dbl, element #3=w381:dbl)  [unwired: 2 in]
        n119 = call <vilib>:"compatOverwrite.vi"("overwrite (F)"=TRUE) -> ("overwrite?"=w354:T7)
        n120 = Bundle By Name(cluster=w379, "Drain Start"=w383, "Drain Stop"=w382, "Drain Step"=w381, "Drain Compliance"=w399, "Range mode"=w362, "Range"=w365) -> (w418:T4)
        n121 = call <userlib>:"4155C Output.vi"("VISA resource name in"=w368, "Gate"=w419, "Drain"=w418, "Timings"=w397, "error in (no error)"=w367, "SMU4"=w356, "sweep mode"=w389, "Panel controls"=w420) -> ("VD"=w406:dbl[], "Outparams"=w359:T8, "VISA Resource Name out"=w395:refnum<visa-resource-name>, "IS"=w409:dbl[], "ID"=w408:dbl[], "IG"=w407:dbl[], "error out"=w396:errorcluster, "SMU4"=w355:dbl[])  [unwired: 12 in]
        n122 = Unbundle By Name(w359) -> ("V2 Step"=w360:dbl, "V2 Start"=w358:dbl, "Number of points"=w357:i32)
        n123 = Open/Create/Replace File(file path (use dialog)=w400, error in=w396, operation (0:open)=w354) -> (refnum out=w415:refnum<file>, error out=w416:errorcluster)  [unwired: 3 in, 1 out]
        n124 = call <userlib>:"4155C Make Big 2d array.vi"("1D Var1"=w406, "1d IS"=w409, "1d ID"=w408, "1d IG"=w407, "1d SMU4"=w355, "SMU4"=w356, "VAR2 START"=w358, "Number of VAR2 steps"=w357, "VAR2 STEP"=w360, "VAR1 Name"="Vd", "Decimal places in header"=i8 1, "VAR2 Name"="Vg") -> ("Header array"=w411:string[], "Data array"=w412:dbl[][])  [unwired: 14 in]
        n125 = call <userlib>:"4155C Write array to file.vi"("Byte Stream File Refnum"=w415, "Header"=w411, "Data Array"=w412, "error in (no error)"=w416) -> ("dup refnum"=w413:refnum<file>, "error out"=w414:errorcluster)  [unwired: 1 in]
        n126 = Close File(refnum=w413, error in=w414) -> (error out=w394:errorcluster)  [unwired: 1 out]
      }
      frame "output-fpp" {
        n127 = Number To Decimal String(number=w475) -> (decimal integer string=w476:string)  [unwired: 1 in]
        n128 = Bundle By Name(cluster=w451, "Emergency Stop"=w479) -> (w489:T6)
        n129 = Delete From Array(array=w466, index=0 ("Index")) -> (deleted portion=w464:string, array with subset deleted=w463:string[])  [unwired: 1 in]
        n130 = Concatenate Strings(w474, "-outputfpp-" ("Substring"), w476, ".txt" ("Substring")) -> (w478:string)
        n131 = VISA Write(VISA resource name=w442, write buffer=":PAGE:CHAN:MODE SWE;" ("write buffer (\"\")"), error in (no error)=w439) -> (VISA resource name out=w441:refnum<visa-resource-name>, error out=w440:errorcluster)  [unwired: 1 out]
        n132 = String To Path(string=w478) -> (path=w473:path)
        n133 = case shown="\"d\", Default" w464 {
          tunnel: [w490 w491] -> w462
          frame "s" {
            w490 = u16 0 items=["Single", "Double"] ("sweep mode")
          }
          frame "d", Default {
            w491 = u16 1 items=["Single", "Double"] ("sweep mode")
          }
        }
        n134 = Fract/Exp String To Number(string=w463) -> (number=w445:dbl[])  [unwired: 3 in, 1 out]
        n135 = Index Array(array=w445, index #1=0 ("Index")) -> (element #1=w461:dbl, element #2=w460:dbl, element #3=w459:dbl)  [unwired: 2 in]
        n136 = Delete From Array(array=w445, length=3 ("Length"), index=0 ("Index")) -> (array with subset deleted=w444:dbl[])  [unwired: 1 out]
        n137 = Bundle By Name(cluster=w453, "Gate Start"=w461, "Gate Stop"=w460, "Gate Step (linear only)"=w459, "Gate Compliance"=w471, "Range mode"=w437, "Range"=w436) -> (w488:T3)
        n138 = Index Array(array=w444, index #1=0 ("Index")) -> (element #1=w456:dbl, element #2=w455:dbl, element #3=w454:dbl)  [unwired: 2 in]
        n139 = call <vilib>:"compatOverwrite.vi"("overwrite (F)"=TRUE) -> ("overwrite?"=w424:T7)
        n140 = Bundle By Name(cluster=w452, "Drain Start"=w456, "Drain Stop"=w455, "Drain Step"=w454, "Drain Compliance"=w472, "Range mode"=w435, "Range"=w438) -> (w487:T4)
        n141 = call <userlib>:"4155C Output-FPP.vi"("VISA resource name in"=w441, "Gate"=w488, "Drain"=w487, "Timings"=w470, "error in (no error)"=w440, "sweep mode"=w462, "Panel controls"=w489) -> ("VD"=w429:dbl[], "Outparams"=w432:T8, "VISA Resource Name out"=w468:refnum<visa-resource-name>, "Vprobe2"=w428:dbl[], "ID"=w427:dbl[], "IG"=w426:dbl[], "Vprobe1"=w425:dbl[], "error out"=w469:errorcluster)  [unwired: 13 in]
        n142 = Unbundle By Name(w432) -> ("V2 Step"=w433:dbl, "V2 Start"=w431:dbl, "Number of points"=w430:i32)
        n143 = Open/Create/Replace File(file path (use dialog)=w473, error in=w469, operation (0:open)=w424) -> (refnum out=w484:refnum<file>, error out=w485:errorcluster)  [unwired: 3 in, 1 out]
        n144 = call <userlib>:"4155C Make Big 2d array FPP.vi"("1D Var1"=w429, "1d ID"=w427, "1d Vp2"=w428, "1d IG"=w426, "1d Vp1"=w425, "VAR2 START"=w431, "Number of VAR2 steps"=w430, "VAR2 STEP"=w433, "VAR1 Name"="Vd", "Decimal places in header"=i8 1, "VAR2 Name"="Vg") -> ("Header array"=w480:string[], "Data array"=w481:dbl[][])  [unwired: 15 in]
        n145 = call <userlib>:"4155C Write array to file.vi"("Byte Stream File Refnum"=w484, "Header"=w480, "Data Array"=w481, "error in (no error)"=w485) -> ("dup refnum"=w482:refnum<file>, "error out"=w483:errorcluster)  [unwired: 1 in]
        n146 = Close File(refnum=w482, error in=w483) -> (error out=w467:errorcluster)  [unwired: 1 out]
      }
      frame "itime" {
        n147 = Delete From Array(array=w504, index=0 ("Index")) -> (deleted portion=w505:string)  [unwired: 1 in, 1 out]
        n148 = case shown="\"l\"" w505 {
          tunnel: w503 -> [w509 w511 w514]
          tunnel: [w508 w510 w513] -> w496
          frame "s" {
            w507 = u32 0 items=["short  ", "medium  ", "long  "] ("integration time 2")
            n149 = Bundle By Name(cluster=w509, "integration time"=w507) -> (w508:T5)
          }
          frame "m", Default {
            w512 = u32 1 items=["short  ", "medium  ", "long  "] ("integration time 2")
            n150 = Bundle By Name(cluster=w511, "integration time"=w512) -> (w510:T5)
          }
          frame "l" {
            w515 = u32 2 items=["short  ", "medium  ", "long  "] ("integration time 2")
            n151 = Bundle By Name(cluster=w514, "integration time"=w515) -> (w513:T5)
          }
        }
      }
      frame "pulsed" {
        n152 = Delete From Array(array=w529, index=0 ("Index")) -> (deleted portion=w530:string, array with subset deleted=w517:string[])  [unwired: 1 in]
        n153 = case shown="\"on\", Default" w530 {
          tunnel: w528 -> [w540 w543]
          tunnel: [w539 w542] -> w521
          tunnel: w517 -> [w537 _]
          frame "on", Default {
            w538 = u16 1 items=["Continuous", "Pulsed"] ("sweep method")
            n154 = Fract/Exp String To Number(string=w537) -> (number=w535:dbl[])  [unwired: 3 in, 1 out]
            n155 = Index Array(array=w535, index #1=0 ("Index")) -> (element #1=w534:dbl, element #2=w533:dbl, element #3=w532:dbl)  [unwired: 2 in]
            n156 = Bundle By Name(cluster=w540, "sweep method"=w538, "Pulse period"=w534, "Base voltage"=w533, "Pulse width"=w532) -> (w539:T5)
          }
          frame "off" {
            w541 = u16 0 items=["Continuous", "Pulsed"] ("sweep method")
            n157 = Bundle By Name(cluster=w543, "sweep method"=w541) -> (w542:T5)
          }
        }
      }
      frame "gaterangemode" {
        n158 = Delete From Array(array=w555, index=0 ("Index")) -> (deleted portion=w556:string)  [unwired: 1 in, 1 out]
        n159 = case shown="\"f\"" w556 {
          tunnel: [w558 w559 w560] -> w545
          frame "a", Default {
            w558 = u16 0 items=["Auto", "Limited", "Fixed"] ("Gate Range\nmode 2")
          }
          frame "f" {
            w559 = u16 2 items=["Auto", "Limited", "Fixed"] ("Gate Range\nmode 2")
          }
          frame "l" {
            w560 = u16 1 items=["Auto", "Limited", "Fixed"] ("Gate Range\nmode 2")
          }
        }
      }
      frame "gaterange" {
        (unwired) u8 11 items=["10fA  ", "100fA  ", "1nA  ", "10nA", "100nA", "1uA", "10uA", "100uA", "1mA", "10mA", "100mA", "1A"] ("Gate Range 2")
        n160 = Delete From Array(array=w579, index=0 ("Index")) -> (deleted portion=w569:string)  [unwired: 1 in, 1 out]
        n161 = Scan Value(string=w569, format string="") -> (value=w567:dbl)  [unwired: 1 in, 1 out]
        n162 = Logarithm Base 10(1:w567) -> (0:w566:dbl)
        n163 = Round To Nearest(number=w566) -> (nearest integer value=w565:dbl)
        n164 = Add(x=w565, y=11.0) -> (x+y=w563:dbl)
        n165 = To Unsigned Byte Integer(number=w563) -> (unsigned 8bit integer=w562:u8)
      }
      frame "drainrange" {
        (unwired) u8 11 items=["10fA  ", "100fA  ", "1nA  ", "10nA", "100nA", "1uA", "10uA", "100uA", "1mA", "10mA", "100mA", "1A"] ("Gate Range 2")
        n166 = Delete From Array(array=w599, index=0 ("Index")) -> (deleted portion=w590:string)  [unwired: 1 in, 1 out]
        n167 = Scan Value(string=w590, format string="") -> (value=w588:dbl)  [unwired: 1 in, 1 out]
        n168 = Logarithm Base 10(1:w588) -> (0:w587:dbl)
        n169 = Round To Nearest(number=w587) -> (nearest integer value=w586:dbl)
        n170 = Add(x=w586, y=11.0) -> (x+y=w584:dbl)
        n171 = To Unsigned Byte Integer(number=w584) -> (unsigned 8bit integer=w583:u8)
      }
      frame "drainrangemode" {
        n172 = Delete From Array(array=w612, index=0 ("Index")) -> (deleted portion=w613:string)  [unwired: 1 in, 1 out]
        n173 = case shown="\"f\"" w613 {
          tunnel: [w615 w616 w617] -> w602
          frame "a", Default {
            w615 = u16 0 items=["Auto", "Limited", "Fixed"] ("Gate Range\nmode 2")
          }
          frame "f" {
            w616 = u16 2 items=["Auto", "Limited", "Fixed"] ("Gate Range\nmode 2")
          }
          frame "l" {
            w617 = u16 1 items=["Auto", "Limited", "Fixed"] ("Gate Range\nmode 2")
          }
        }
      }
      frame "Error", Default {
      }
      frame "logfile" {
        n174 = Number To Decimal String(number=w660) -> (decimal integer string=w664:string)  [unwired: 1 in]
        n175 = Concatenate Strings(w662, "logfile" ("Substring"), w664, ".txt" ("Substring")) -> (w659:string)
        n176 = String To Path(string=w659) -> (path=w632:path)
        n177 = Unbundle(w658) -> ("integration time"=w657:u32, "Short/Long integration time"=w656:dbl, "hold time (sec)"=w655:dbl, "delay time (sec)"=w654:dbl, "Step Time (0 disables)"=w653:dbl, "sweep method"=w652:u16, "Pulse period"=w651:dbl, "Base voltage"=w650:dbl, "Pulse width"=w649:dbl)
        n178 = Build Array(w657, w656, w655, w654, w653, w652, w651, w650, w649, w643, w644, w645, w646, w647, w648) -> (w636:dbl[])
        n179 = Insert Into Array(array=dbl[][] [] ("Input Array"), new element=w636) -> (w635:dbl[][])  [unwired: 2 in]
        n180 = call <vilib>:"compatOverwrite.vi"("overwrite (F)"=TRUE) -> ("overwrite?"=w630:T7)
        n181 = Open/Create/Replace File(file path (use dialog)=w632, error in=w634, operation (0:open)=w630) -> (refnum out=w640:refnum<file>, error out=w639:errorcluster)  [unwired: 3 in, 1 out]
        n182 = call <userlib>:"4155C Write array to file.vi"("Byte Stream File Refnum"=w640, "Header"=string[] ["Int Time", "Short/Long Itime", "Hold time", "Delay time", "Step time", "Sweep method", "Pulse period", "Base Voltage", "Pulse width", "Drain compliance", "Gate compliance", "Gate range mode", "Gate range", "S/D range mode", "S/D range"], "Data Array"=w635, "error in (no error)"=w639) -> ("dup refnum"=w642:refnum<file>, "error out"=w641:errorcluster)  [unwired: 1 in]
        n183 = Close File(refnum=w642, error in=w641) -> (error out=w633:errorcluster)  [unwired: 1 out]
      }
      frame "sample" {
        n184 = Number To Decimal String(number=w714) -> (decimal integer string=w713:string)  [unwired: 1 in]
        n185 = Fract/Exp String To Number(string=w710) -> (number=w670:dbl[])  [unwired: 3 in, 1 out]
        n186 = Concatenate Strings(w688, "-sample-" ("Substring"), w713, ".txt" ("Substring")) -> (w711:string)
        n187 = String To Path(string=w711) -> (path=w692:path)
        n188 = Index Array(array=w670, index=0 ("Index")) -> (element=w708:dbl)
        n189 = Index Array(array=w670, index=2 ("Index")) -> (element=w704:dbl)
        n190 = Index Array(array=w670, index=3 ("Index")) -> (element=w673:dbl)
        n191 = Index Array(array=w670, index=4 ("Index")) -> (element=w669:dbl)
        n192 = call <userlib>:"4155C Config Sampling Measurements.vi"("Sampling interval"=w669, "Sample time"=w673, "Display on/off"=TRUE, "Timings"=w679, "Num Points"=w704, "error in (no error)"=w716, "Drain Compliance"=w715, "Gate Compliance"=w689, "VISA session"=w717) -> ("error out"=w718:errorcluster, "dup VISA resource name"=w719:refnum<visa-resource-name>)  [unwired: 1 in]
        n193 = Index Array(array=w670, index=1 ("Index")) -> (element=w705:dbl)
        n194 = call <userlib>:"4155C Take Sample.vi"("Emergency Stop"=w685, "error in (no error)"=w718, "Vd"=w705, "Vg"=w708, "VISA resource name in"=w719) -> ("error out"=w683:errorcluster, "Id"=w721:dbl[], "Ig"=w694:dbl[], "VISA Resource Name out"=w681:refnum<visa-resource-name>, "Is"=w720:dbl[], "Time"=w698:dbl[])  [unwired: 1 in]
        n195 = Insert Into Array(array=dbl[][] [] ("Input Array"), new element=w698) -> (w697:dbl[][])  [unwired: 2 in]
        n196 = Insert Into Array(array=w697, new element=w694) -> (w696:dbl[][])  [unwired: 2 in]
        n197 = Insert Into Array(array=w696, new element=w721) -> (w695:dbl[][])  [unwired: 2 in]
        n198 = VISA Write(VISA resource name=w681, write buffer=":DISP ON" ("write buffer (\"\")"), error in (no error)=w683) -> (VISA resource name out=w680:refnum<visa-resource-name>, error out=w682:errorcluster)  [unwired: 1 out]
        n199 = Insert Into Array(array=w695, new element=w720) -> (w687:dbl[][])  [unwired: 2 in]
        n200 = Transpose 2D Array(2D array=w687) -> (transposed array=w686:dbl[][])
        n201 = call <vilib>:"compatOverwrite.vi"("overwrite (F)"=TRUE) -> ("overwrite?"=w667:T7)
        n202 = Open/Create/Replace File(file path (use dialog)=w692, error in=w682, operation (0:open)=w667) -> (refnum out=w701:refnum<file>, error out=w700:errorcluster)  [unwired: 3 in, 1 out]
        n203 = call <userlib>:"4155C Write array to file.vi"("Byte Stream File Refnum"=w701, "Header"=string[] ["Time /s", "Ig /A", "Id /A", "Is /A"], "Data Array"=w686, "error in (no error)"=w700) -> ("dup refnum"=w703:refnum<file>, "error out"=w702:errorcluster)  [unwired: 1 in]
        n204 = Close File(refnum=w703, error in=w702) -> (error out=w690:errorcluster)  [unwired: 1 out]
      }
      frame "samplei" {
        n205 = Number To Decimal String(number=w773) -> (decimal integer string=w772:string)  [unwired: 1 in]
        n206 = Fract/Exp String To Number(string=w769) -> (number=w735:dbl[])  [unwired: 3 in, 1 out]
        n207 = Concatenate Strings(w751, "-samplei-" ("Substring"), w772, ".txt" ("Substring")) -> (w770:string)
        n208 = String To Path(string=w770) -> (path=w754:path)
        n209 = Index Array(array=w735, index=4 ("Index")) -> (element=w729:dbl)
        n210 = Index Array(array=w735, index=3 ("Index")) -> (element=w730:dbl)
        n211 = Index Array(array=w735, index=1 ("Index")) -> (element=w732:dbl)
        n212 = Index Array(array=w735, index=0 ("Index")) -> (element=w733:dbl)
        n213 = Index Array(array=w735, index=2 ("Index")) -> (element=w731:dbl)
        n214 = call <userlib>:"4155C Config SamplingI Measurements.vi"("Sample time"=w731, "Display on/off"=TRUE, "Timings"=w743, "Num Points"=w732, "error in (no error)"=w775, "Sampling interval"=w730, "VISA session"=w776) -> ("error out"=w777:errorcluster, "dup VISA resource name"=w778:refnum<visa-resource-name>)  [unwired: 3 in]
        n215 = call <userlib>:"4155C Take SampleI.vi"("Emergency Stop"=w748, "error in (no error)"=w777, "Idg 2"=w733, "Vdg compliance 2"=w729, "VISA resource name in"=w778) -> ("error out"=w746:errorcluster, "Idg"=w780:dbl[], "Vdg"=w756:dbl[], "VISA Resource Name out"=w744:refnum<visa-resource-name>, "Is"=w779:dbl[], "Time"=w760:dbl[])  [unwired: 1 in]
        n216 = Insert Into Array(array=dbl[][] [] ("Input Array"), new element=w760) -> (w759:dbl[][])  [unwired: 2 in]
        n217 = Insert Into Array(array=w759, new element=w756) -> (w758:dbl[][])  [unwired: 2 in]
        n218 = Insert Into Array(array=w758, new element=w780) -> (w757:dbl[][])  [unwired: 2 in]
        n219 = VISA Write(VISA resource name=w744, write buffer=":DISP ON" ("write buffer (\"\")"), error in (no error)=w746) -> (VISA resource name out=w728:refnum<visa-resource-name>, error out=w745:errorcluster)  [unwired: 1 out]
        n220 = Insert Into Array(array=w757, new element=w779) -> (w750:dbl[][])  [unwired: 2 in]
        n221 = Transpose 2D Array(2D array=w750) -> (transposed array=w749:dbl[][])
        n222 = call <vilib>:"compatOverwrite.vi"("overwrite (F)"=TRUE) -> ("overwrite?"=w723:T7)
        n223 = Open/Create/Replace File(file path (use dialog)=w754, error in=w745, operation (0:open)=w723) -> (refnum out=w763:refnum<file>, error out=w762:errorcluster)  [unwired: 3 in, 1 out]
        n224 = call <userlib>:"4155C Write array to file.vi"("Byte Stream File Refnum"=w763, "Header"=string[] ["Time /s", "Vdg /V", "Idg /A", "Is /A"], "Data Array"=w749, "error in (no error)"=w762) -> ("dup refnum"=w765:refnum<file>, "error out"=w764:errorcluster)  [unwired: 1 in]
        n225 = Close File(refnum=w765, error in=w764) -> (error out=w726:errorcluster)  [unwired: 1 out]
        n226 = VISA Write(VISA resource name=w728, write buffer=";:PAGE:SCON:STAN OFF;:PAGE:CHAN:VSU2:DIS;" ("write buffer (\"\")"), error in (no error)=w726) -> (VISA resource name out=w724:refnum<visa-resource-name>, error out=w725:errorcluster)  [unwired: 1 out]
      }
      frame "#" {
        n227 = VISA Write(VISA resource name=w786, write buffer=":DISP ON" ("write buffer (\"\")"), error in (no error)=w785) -> (VISA resource name out=w784:refnum<visa-resource-name>, error out=w783:errorcluster)  [unwired: 1 out]
      }
      frame "stressV" {
        n228 = Number To Decimal String(number=w835) -> (decimal integer string=w834:string)  [unwired: 1 in]
        n229 = Fract/Exp String To Number(string=w831) -> (number=w803:dbl[])  [unwired: 3 in, 1 out]
        n230 = Concatenate Strings(w818, "-stressV-" ("Substring"), w834, ".txt" ("Substring")) -> (w832:string)
        n231 = String To Path(string=w832) -> (path=w822:path)
        n232 = Index Array(array=w803, index=3 ("Index")) -> (element=w800:dbl)
        n233 = Index Array(array=w803, index=1 ("Index")) -> (element=w798:dbl)
        n234 = Index Array(array=w803, index=0 ("Index")) -> (element=w797:dbl)
        n235 = Index Array(array=w803, index=4 ("Index")) -> (element=w802:dbl)
        n236 = Index Array(array=w803, index=2 ("Index")) -> (element=w799:dbl)
        n237 = call <userlib>:"4155C Config V Stress.vi"("VISA session"=w838, "ID compliance"=w800, "VD"=w798, "VG"=w797, "IG compliance"=w799, "error in (no error)"=w837, "Display on/off"=TRUE) -> ("dup VISA resource name"=w840:refnum<visa-resource-name>, "error out"=w839:errorcluster)
        n238 = call <userlib>:"4155C Apply Stress.vi"("error in (no error)"=w839, "Duration"=w802, "Emergency Stop"=w817, "VISA resource name in"=w840) -> ("error out"=w815:errorcluster, "VISA Resource Name out"=w813:refnum<visa-resource-name>)
        n239 = VISA Write(VISA resource name=w813, write buffer=":DISP ON" ("write buffer (\"\")"), error in (no error)=w815) -> (VISA resource name out=w812:refnum<visa-resource-name>, error out=w814:errorcluster)  [unwired: 1 out]
        n240 = call <vilib>:"compatOverwrite.vi"("overwrite (F)"=TRUE) -> ("overwrite?"=w796:T7)
        n241 = Open/Create/Replace File(file path (use dialog)=w822, error in=w814, operation (0:open)=w796) -> (refnum out=w825:refnum<file>, error out=w824:errorcluster)  [unwired: 3 in, 1 out]
        n242 = call <userlib>:"4155C Write array to file.vi"("Byte Stream File Refnum"=w825, "Header"=string[] ["V stress completed successfully", ""], "error in (no error)"=w824) -> ("dup refnum"=w827:refnum<file>, "error out"=w826:errorcluster)  [unwired: 2 in]
        n243 = Close File(refnum=w827, error in=w826) -> (error out=w820:errorcluster)  [unwired: 1 out]
      }
      frame "stressI" {
        n244 = Number To Decimal String(number=w877) -> (decimal integer string=w876:string)  [unwired: 1 in]
        n245 = Fract/Exp String To Number(string=w873) -> (number=w847:dbl[])  [unwired: 3 in, 1 out]
        n246 = Concatenate Strings(w860, "-stressI-" ("Substring"), w876, ".txt" ("Substring")) -> (w874:string)
        n247 = String To Path(string=w874) -> (path=w864:path)
        n248 = Index Array(array=w847, index=1 ("Index")) -> (element=w843:dbl)
        n249 = Index Array(array=w847, index=0 ("Index")) -> (element=w844:dbl)
        n250 = call <userlib>:"4155C Config I Stress.vi"("VISA session"=w880, "IDG"=w844, "VDG compliance"=w843, "error in (no error)"=w879, "Display on/off"=TRUE) -> ("dup VISA resource name"=w882:refnum<visa-resource-name>, "error out"=w881:errorcluster)
        n251 = Index Array(array=w847, index=2 ("Index")) -> (element=w845:dbl)
        n252 = call <userlib>:"4155C Apply Stress.vi"("error in (no error)"=w881, "Duration"=w845, "Emergency Stop"=w859, "VISA resource name in"=w882) -> ("error out"=w857:errorcluster, "VISA Resource Name out"=w855:refnum<visa-resource-name>)
        n253 = VISA Write(VISA resource name=w855, write buffer=":DISP ON" ("write buffer (\"\")"), error in (no error)=w857) -> (VISA resource name out=w854:refnum<visa-resource-name>, error out=w856:errorcluster)  [unwired: 1 out]
        n254 = call <vilib>:"compatOverwrite.vi"("overwrite (F)"=TRUE) -> ("overwrite?"=w842:T7)
        n255 = Open/Create/Replace File(file path (use dialog)=w864, error in=w856, operation (0:open)=w842) -> (refnum out=w867:refnum<file>, error out=w866:errorcluster)  [unwired: 3 in, 1 out]
        n256 = call <userlib>:"4155C Write array to file.vi"("Byte Stream File Refnum"=w867, "Header"=string[] ["I stress completed successfully", ""], "error in (no error)"=w866) -> ("dup refnum"=w869:refnum<file>, "error out"=w868:errorcluster)  [unwired: 2 in]
        n257 = Close File(refnum=w869, error in=w868) -> (error out=w862:errorcluster)  [unwired: 1 out]
      }
      frame "vsu2pulse" {
        n258 = Number To Decimal String(number=w917) -> (decimal integer string=w916:string)  [unwired: 1 in]
        n259 = Fract/Exp String To Number(string=w913) -> (number=w888:dbl[])  [unwired: 3 in, 1 out]
        n260 = Concatenate Strings(w901, "-vsu2-" ("Substring"), w916, ".txt" ("Substring")) -> (w914:string)
        n261 = String To Path(string=w914) -> (path=w905:path)
        n262 = Index Array(array=w888, index=1 ("Index")) -> (element=w887:dbl)
        n263 = Index Array(array=w888, index=0 ("Index")) -> (element=w885:dbl)
        n264 = call <userlib>:"4155C Config VSU2 Stress.vi"("error in (no error)"=w919, "VSU2"=w885, "Display on/off"=TRUE, "VISA session"=w920) -> ("error out"=w921:errorcluster, "dup VISA resource name"=w922:refnum<visa-resource-name>)
        n265 = call <userlib>:"4155C Apply Stress.vi"("error in (no error)"=w921, "Duration"=w887, "Emergency Stop"=w900, "VISA resource name in"=w922) -> ("error out"=w898:errorcluster, "VISA Resource Name out"=w896:refnum<visa-resource-name>)
        n266 = VISA Write(VISA resource name=w896, write buffer=":DISP ON" ("write buffer (\"\")"), error in (no error)=w898) -> (VISA resource name out=w895:refnum<visa-resource-name>, error out=w897:errorcluster)  [unwired: 1 out]
        n267 = call <vilib>:"compatOverwrite.vi"("overwrite (F)"=TRUE) -> ("overwrite?"=w884:T7)
        n268 = Open/Create/Replace File(file path (use dialog)=w905, error in=w897, operation (0:open)=w884) -> (refnum out=w908:refnum<file>, error out=w907:errorcluster)  [unwired: 3 in, 1 out]
        n269 = call <userlib>:"4155C Write array to file.vi"("Byte Stream File Refnum"=w908, "Header"=string[] ["VSU2 pulse completed successfully", ""], "error in (no error)"=w907) -> ("dup refnum"=w910:refnum<file>, "error out"=w909:errorcluster)  [unwired: 2 in]
        n270 = Close File(refnum=w910, error in=w909) -> (error out=w903:errorcluster)  [unwired: 1 out]
      }
      frame "sample-fpp" {
        w931 = string[] ["Time /s", "Id VgVd /A", "Ig VgVd /A", "Vp1 VgVd /V", "Vp2 VgVd /V"] ("Header")
        w935 = "%d" ("format string")
        n271 = Number To Decimal String(number=w985) -> (decimal integer string=w984:string)  [unwired: 1 in]
        n272 = Fract/Exp String To Number(string=w981) -> (number=w969:dbl[])  [unwired: 3 in, 1 out]
        n273 = Concatenate Strings(w975, "-samplefpp-" ("Substring"), w984, ".txt" ("Substring")) -> (w982:string)
        n274 = String To Path(string=w982) -> (path=w943:path)
        n275 = Index Array(array=w969, index=0 ("Index")) -> (element=w929:dbl)
        n276 = Index Array(array=w969, index=1 ("Index")) -> (element=w928:dbl)
        n277 = Index Array(array=w969, index=2 ("Index")) -> (element=w977:dbl)
        n278 = Index Array(array=w969, index=3 ("Index")) -> (element=w967:dbl)
        n279 = call <userlib>:"4155C Config Sampling Measurements FPP.vi"("VISA session"=w988, "Num Points"=w977, "Vg"=w929, "Display on/off"=TRUE, "Gate Compliance"=w976, "Drain Compliance"=w986, "Standby"="Standby", "error in (no error)"=w987, "Timings"=w974, "Vd"=w928, "Sample time"=w967) -> ("dup VISA resource name"=w945:refnum<visa-resource-name>, "error out"=w944:errorcluster)  [unwired: 3 in]
        n280 = Number To Decimal String(number=w929) -> (decimal integer string=w955:string)  [unwired: 1 in]
        n281 = call <userlib>:"4155C Take Sample FPP.vi"("VISA resource name in"=w945, "error in (no error)"=w944, "Emergency Stop"=w946) -> ("Time"=w950:dbl[], "Vp1"=w960:dbl[], "VISA Resource Name out"=w926:refnum<visa-resource-name>, "Ig"=w948:dbl[], "Id"=w949:dbl[], "Vp2"=w958:dbl[], "error out"=w947:errorcluster)  [unwired: 10 in]
        n282 = Insert Into Array(array=dbl[][] [] ("Input Array"), new element=w950) -> (w964:dbl[][])  [unwired: 2 in]
        n283 = Number To Decimal String(number=w928) -> (decimal integer string=w953:string)  [unwired: 1 in]
        n284 = Insert Into Array(array=w964, new element=w949) -> (w963:dbl[][])  [unwired: 2 in]
        n285 = Concatenate Strings("(Vg = " ("Substring"), w955, "V, Vd = " ("Substring"), w953, "V)" ("Substring")) -> (w951:string)
        n286 = Insert Into Array(array=w963, new element=w948) -> (w962:dbl[][])  [unwired: 2 in]
        n287 = Insert Into Array(array=w962, new element=w960) -> (w959:dbl[][])  [unwired: 2 in]
        n288 = Insert Into Array(array=w959, new element=w958) -> (w927:dbl[][])  [unwired: 2 in]
        n289 = call <vilib>:"compatOverwrite.vi"("overwrite (F)"=TRUE) -> ("overwrite?"=w924:T7)
        n290 = Open/Create/Replace File(file path (use dialog)=w943, error in=w947, operation (0:open)=w924) -> (refnum out=w940:refnum<file>, error out=w941:errorcluster)  [unwired: 3 in, 1 out]
        n291 = Array To Spreadsheet String(array=w931, 3:w935) -> (spreadsheet string=w937:string)  [unwired: 1 in]
        n292 = Transpose 2D Array(2D array=w927) -> (transposed array=w957:dbl[][])
        n293 = Search and Replace String(replace all?=TRUE ("replace all? (F)"), input string=w937, search string="VgVd", replace string=w951) -> (result string=w933:string)  [unwired: 4 in, 3 out]
        n294 = Spreadsheet String To Array(format string=w935, spreadsheet string=w933, array type (2D Dbl)=w931) -> (array=w932:string[])  [unwired: 1 in]
        n295 = call <userlib>:"4155C Write array to file.vi"("Byte Stream File Refnum"=w940, "Header"=w932, "Data Array"=w957, "error in (no error)"=w941) -> ("dup refnum"=w938:refnum<file>, "error out"=w939:errorcluster)  [unwired: 1 in]
        n296 = Close File(refnum=w938, error in=w939) -> (error out=w925:errorcluster)  [unwired: 1 out]
      }
      frame "resample-fpp" {
        w999 = string[] ["Time /s", "Id VgVd /A", "Ig VgVd /A", "Vp1 VgVd /V", "Vp2 VgVd /V"] ("Header")
        w1003 = "%d" ("format string")
        n297 = Number To Decimal String(number=w1045) -> (decimal integer string=w1044:string)  [unwired: 1 in]
        n298 = Fract/Exp String To Number(string=w1041) -> (number=w992:dbl[])  [unwired: 3 in, 1 out]
        n299 = Concatenate Strings(w1037, "-resamplefpp-" ("Substring"), w1044, ".txt" ("Substring")) -> (w1042:string)
        n300 = String To Path(string=w1042) -> (path=w1011:path)
        n301 = Index Array(array=w992, index=0 ("Index")) -> (element=w998:dbl)
        n302 = Index Array(array=w992, index=1 ("Index")) -> (element=w997:dbl)
        n303 = Number To Decimal String(number=w998) -> (decimal integer string=w1021:string)  [unwired: 1 in]
        n304 = call <userlib>:"4155C Take Sample FPP.vi"("VISA resource name in"=w994, "error in (no error)"=w993, "Emergency Stop"=w1012) -> ("Time"=w1016:dbl[], "Vp1"=w1026:dbl[], "VISA Resource Name out"=w996:refnum<visa-resource-name>, "Ig"=w1014:dbl[], "Id"=w1015:dbl[], "Vp2"=w1024:dbl[], "error out"=w1013:errorcluster)  [unwired: 10 in]
        n305 = Insert Into Array(array=dbl[][] [] ("Input Array"), new element=w1016) -> (w1030:dbl[][])  [unwired: 2 in]
        n306 = Number To Decimal String(number=w997) -> (decimal integer string=w1019:string)  [unwired: 1 in]
        n307 = Insert Into Array(array=w1030, new element=w1015) -> (w1029:dbl[][])  [unwired: 2 in]
        n308 = Concatenate Strings("(Vg = " ("Substring"), w1021, "V, Vd = " ("Substring"), w1019, "V)" ("Substring")) -> (w1017:string)
        n309 = Insert Into Array(array=w1029, new element=w1014) -> (w1028:dbl[][])  [unwired: 2 in]
        n310 = Insert Into Array(array=w1028, new element=w1026) -> (w1025:dbl[][])  [unwired: 2 in]
        n311 = Insert Into Array(array=w1025, new element=w1024) -> (w991:dbl[][])  [unwired: 2 in]
        n312 = call <vilib>:"compatOverwrite.vi"("overwrite (F)"=TRUE) -> ("overwrite?"=w990:T7)
        n313 = Open/Create/Replace File(file path (use dialog)=w1011, error in=w1013, operation (0:open)=w990) -> (refnum out=w1008:refnum<file>, error out=w1009:errorcluster)  [unwired: 3 in, 1 out]
        n314 = Array To Spreadsheet String(array=w999, 3:w1003) -> (spreadsheet string=w1005:string)  [unwired: 1 in]
        n315 = Transpose 2D Array(2D array=w991) -> (transposed array=w1023:dbl[][])
        n316 = Search and Replace String(replace all?=TRUE ("replace all? (F)"), input string=w1005, search string="VgVd", replace string=w1017) -> (result string=w1001:string)  [unwired: 4 in, 3 out]
        n317 = Spreadsheet String To Array(format string=w1003, spreadsheet string=w1001, array type (2D Dbl)=w999) -> (array=w1000:string[])  [unwired: 1 in]
        n318 = call <userlib>:"4155C Write array to file.vi"("Byte Stream File Refnum"=w1008, "Header"=w1000, "Data Array"=w1023, "error in (no error)"=w1009) -> ("dup refnum"=w1006:refnum<file>, "error out"=w1007:errorcluster)  [unwired: 1 in]
        n319 = Close File(refnum=w1006, error in=w1007) -> (error out=w995:errorcluster)  [unwired: 1 out]
      }
    }
    n320 = local write "Lines left to run:"(w41) -> ()
    n321 = Empty String/Path?(string/path=w41) -> (empty?=w77:bool)
    n322 = Not(x=w77) -> (.not. x?=w76:bool)
  }
